vi "Failsafe.vi"(4 "Settings":cluster{"Numeric":dbl, "Boolean":bool}, 6 "Name of Experiment":string, 7 "Danger?":bool, 8 "error in":errorcluster, 9 "Emergency Contact (Carrier)":enum16{"T-Mobile", "AT&T", "Verizon", "Sprint"}(ring), 10 "Emergency Contact (phone number)":string, 11 "Path In":path) -> (0 "error out":errorcluster, 3 "Path Out":path)   [LabVIEW 2018]
uses:
  <vilib>/smtpClient/Set Message Text.vi
  <vilib>/smtpClient/LabVIEWSMTPClient.lvlib
panel:
  in  "TLS":bool=TRUE
  in  "Outgoing Mail Server (SMTP)":string="smtp.gmail.com"
  in  "Body":string="Error"
  in  "Password":string="labVIEW123"
  in  "Email":string="krishna16842@gmail.com"
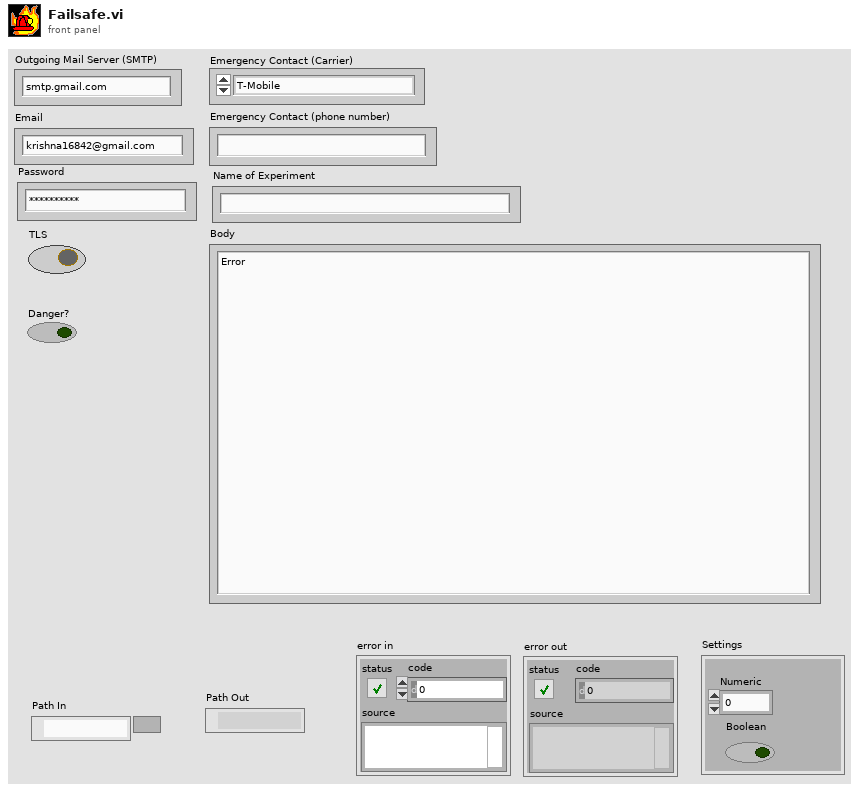
[diagram p1: front panel]
types:
  T1 = typedef "LabVIEWSMTPClient.lvlib/SmtpClientHandle.ctl" = refnum<k1>
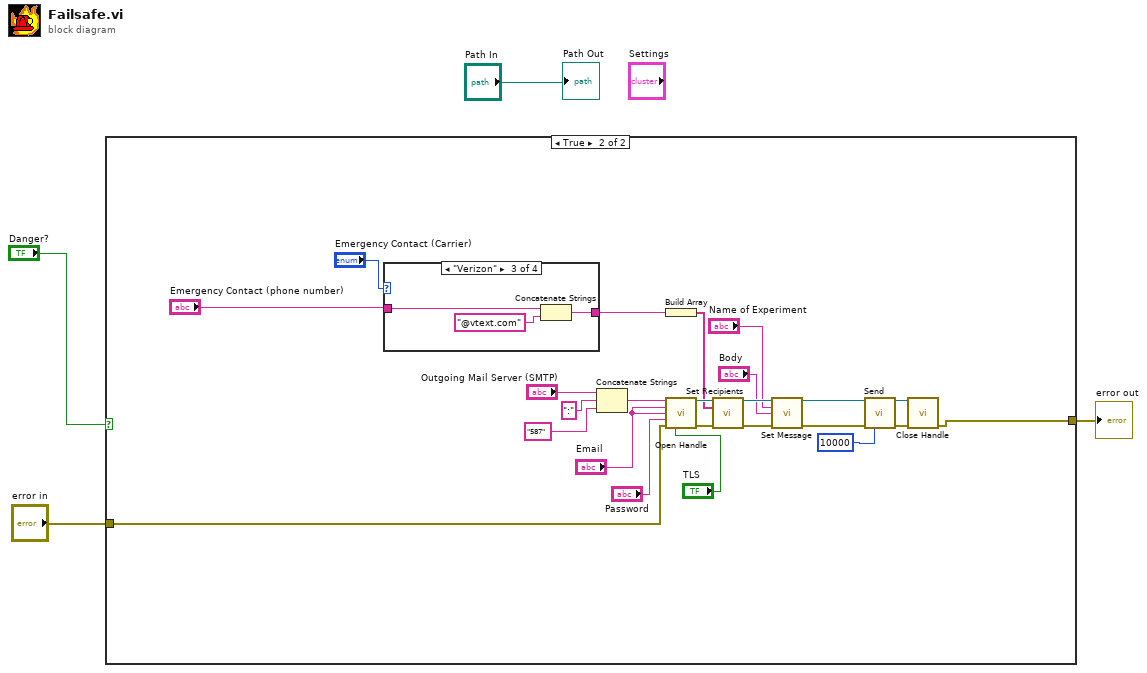
[diagram p0: block diagram]
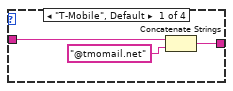
[diagram p3: hidden frame]
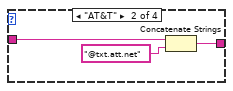
[diagram p4: hidden frame]
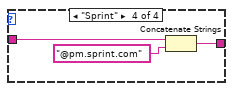
[diagram p5: hidden frame]
diagram:
  n1 = case shown="True" "Danger?" {
    tunnel: "error in" -> [w5 w7]
    tunnel: [w5 w6] -> w2
    frame False {
    }
    frame True {
      n2 = case shown="\"Verizon\"" "Emergency Contact (Carrier)" {
        tunnel: "Emergency Contact (phone number)" -> [w32 w34 w37 w40]
        tunnel: [w30 w35 w38 w41] -> w15
        frame "T-Mobile", Default {
          n3 = Concatenate Strings(w32, "@tmomail.net" ("string")) -> (w30:string)
        }
        frame "AT&T" {
          n4 = Concatenate Strings(w34, "@txt.att.net" ("string")) -> (w35:string)
        }
        frame "Verizon" {
          n5 = Concatenate Strings(w37, "@vtext.com" ("string")) -> (w38:string)
        }
        frame "Sprint" {
          n6 = Concatenate Strings(w40, "@pm.sprint.com") -> (w41:string)
        }
      }
      n7 = Concatenate Strings("Outgoing Mail Server (SMTP)", ":" ("string"), "587" ("Port")) -> (w10:string)
      n8 = Build Array(w15) -> (w14:string[])
      n9 = call <vilib>:"Open Handle.vi"("server address"=w10, "from"="Email", "username"="Email", "password"="Password", "error in (no error)"=w7, "use TLS (false)"="TLS") -> ("handle out"=w27:T1, "error out"=w24:errorcluster)  [unwired: 8 in]
      n10 = call <vilib>:"Set Recipients.vi"("handle in"=w27, "to"=w14, "error in (no error)"=w24) -> ("handle out"=w23:T1, "error out"=w22:errorcluster)  [unwired: 11 in]
      n11 = call-poly <vilib>:"Set Message.vi"("handle in"=w23, "subject"="Name of Experiment", "plain text message"="Body", "error in (no error)"=w22) -> ("handle out"=w19:T1, "error out"=w18:errorcluster)  [unwired: 10 in]
      n12 = call <vilib>:"Send.vi"("handle in"=w19, "error in (no error)"=w18, "timeout in ms (10000)"=10000) -> ("handle out"=w17:T1, "error out"=w16:errorcluster)  [unwired: 10 in, 1 out]
      n13 = call <vilib>:"Close Handle.vi"("handle in"=w17, "error in (no error)"=w16) -> ("error out"=w6:errorcluster)  [unwired: 12 in, 1 out]
    }
  }
  "error out" <- w2
  "Path Out" <- "Path In"
